vi "DigitalIn.vi"(8 "error in (no error)":errorcluster, 9 "Existing Obj Name":string, 10 "Pin":string, 11 "mbed_LVLibrary.lvlib:mbed.lvclass":refnum<class "mbed.lvclass">) -> (0 "error out":errorcluster, 1 "Assigned Name":string, 3 "DigitalIn.lvclass 2":refnum<class "DigitalIn.lvclass">)   [LabVIEW 2011, in "mbed_LVLibrary.lvlib" / "DigitalIn.lvclass"]
doc: "This VI creates a DigitalIn on an mbed pin. It takes either the pin number as a string (eg \"p21\") or the name of an existing DigitalIn object on mbed."
uses:
  DigitalIn.lvclass
  Transport Mechanisms/mbed/mbed.lvclass
  DigitalIn.lvclass/DigitalIn.ctl
  <vilib>/regexp/Match Regular Expression.xnode
panel:
  in  "DigitalIn.lvclass":refnum<class "DigitalIn.lvclass">
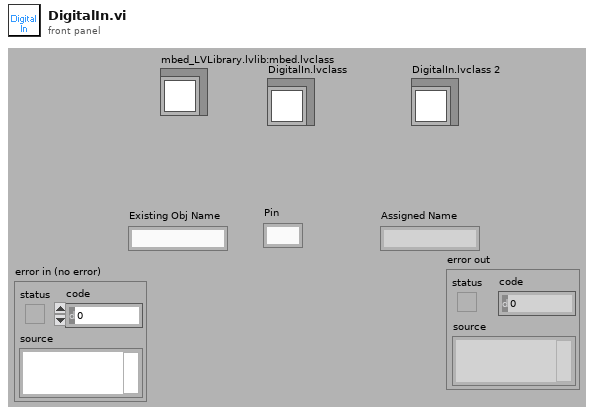
[diagram p1: front panel]
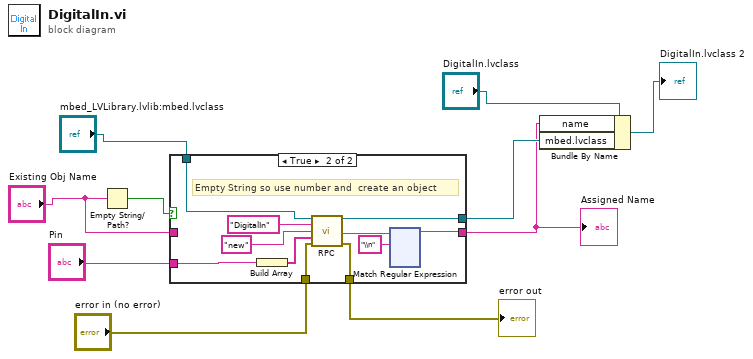
[diagram p0: block diagram]
diagram:
  n1 = Empty String/Path?(string/path="Existing Obj Name") -> (empty?=w7:bool)
  n2 = case shown="True" w7 {
    tunnel: "Existing Obj Name" -> [w13 _]
    tunnel: [w13 w20] -> w8
    tunnel: "mbed_LVLibrary.lvlib:mbed.lvclass" -> [w12 w24]
    tunnel: [w12 w21] -> w9
    tunnel: "Pin" -> [_ w16]
    tunnel: "error in (no error)" -> [w11 w15]
    tunnel: [w11 w14] -> w2
    frame False {
      # "String present so just set the class name"
    }
    frame True {
      # "Empty String so use number and  create an object"
      n3 = Build Array(w16) -> (w17:string[])
      n4 = call-dynamic "RPC.vi"("mbed in"=w24, "Name"="DigitalIn", "method"="new", "Args"=w17, "error in (no error)"=w15) -> ("mbed out"=w21:refnum<class "mbed.lvclass">, "RPC Result"=w19:string, "error out"=w14:errorcluster)  [unwired: 8 in]
      n5 = xnode "Match Regular Expression"("input string"=w19, "regular expression"="\\n") -> ("before match"=w20:string)  [unwired: 4 in, 4 out]
    }
  }
  "Assigned Name" <- w8
  "error out" <- w2
  n6 = Bundle By Name(cluster="DigitalIn.lvclass", "name"=w8, "mbed.lvclass"=w9) -> (→"DigitalIn.lvclass 2":refnum<class "DigitalIn.lvclass">)
